vi "IsValidNode.vi"(10 "Node Name":string, 11 "Server in":refnum<class "Server.lvclass">) -> (2 "Valid Node Definition?":bool, 3 "Server out":refnum<class "Server.lvclass">)   [LabVIEW 2015, in "JKI_Python_Bridge_for_LV.lvlib" / "Server.lvclass"]
uses:
  Server.lvclass
  <userlib>/_OpenG.lib/file/file.llb/Valid Path - Traditional__ogtk.vi
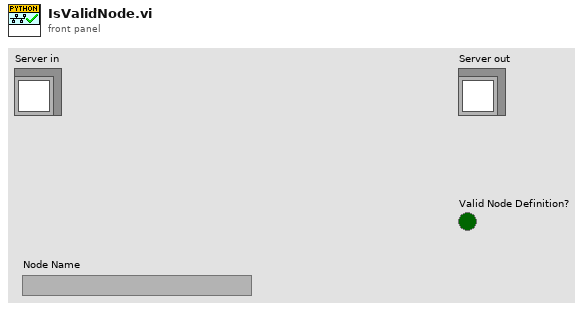
[diagram p1: front panel]
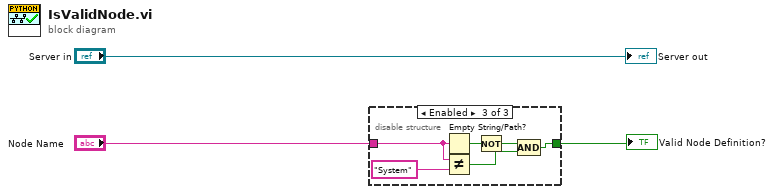
[diagram p0: block diagram]
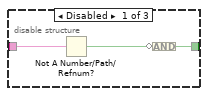
[diagram p2: hidden frame]
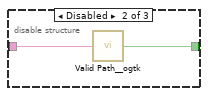
[diagram p3: hidden frame]
diagram:
  n1 = disable-structure shown="Enabled" {
    disable-tunnel: [w6 w7 w10] -> w2
    disable-tunnel: "Node Name" -> [w4 w8 w12]
    frame Disabled {
      n2 = Not A Number/Path/Refnum?(number/path/refnum=w4) -> (NaN/Path/Refnum?=w5:bool)
      n3 = Compound Arithmetic op=AND(invert w5) -> (w6:bool)
    }
    frame Disabled {
      n4 = call-poly <userlib>:"Valid Path__ogtk.vi"("path"=w8) -> ("valid"=w7:bool)
    }
    frame Enabled {
      n5 = Empty String/Path?(string/path=w12) -> (empty?=w14:bool)
      n6 = Not Equal?(x=w12, y="System") -> (x != y?=w9:bool)
      n7 = Not(x=w14) -> (.not. x?=w13:bool)
      n8 = Compound Arithmetic op=AND(w13, w9) -> (w10:bool)
    }
  }
  "Valid Node Definition?" <- w2
  "Server out" <- "Server in"
